vi "Flowmeter_Count and Period.vi"() -> ()   [LabVIEW 2013]
doc: "This VI counts the number of rising edges since the last sample event and measures the total period from the first to last edge in the measurement window. Divide count by period to determine the frequency."
uses:
  <vilib>/Platform/TimedLoop/XDataNode/timing_clust.ctl
  <vilib>/Platform/TimedLoop/XDataNode/nitl_modes.ctl
  <vilib>/Platform/TimedLoop/XDataNode/wakeup.ctl
  <vilib>/rvi/Emulation/niFpgaSctlEmulationGetInTimedLoop.vi
  <vilib>/rvi/Emulation/niFpgaEmulationReportErrorSimple.vi
  <vilib>/rvi/Emulation/niFpgaGetClockAttributes.vi
  <vilib>/rvi/Emulation/niFpgaCriticalErrorInLSC.vi
  <vilib>/rvi/eio/common/nirviEmuTemplateMethod_errors.vi
  Instance           2 31Saved   Count and Period (FPGA) .vi
  <vilib>/Platform/TimedLoop/XDataNode/XDataNode.xnode
  <vilib>/eio/EIONode/EIONode.xnode
  <vilib>/Platform/TimedLoop/XDataNode/XDNodeRunTimeDep.lvlib
panel:
  out "Count":u32
  out "Period":u32
  in  "Sample":bool
  in  "Polarity":bool
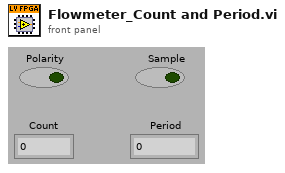
[diagram p1: front panel]
types:
  T1 = typedef "XDNodeRunTimeDep.lvlib/timing_clust.ctl" = cluster{"Expected End [f-1]":u64, "Actual End [f-1]":u64, "Finished Late? [f-1]":bool, "Expected End [i-1]":u64, "Actual End [i-1]":u64, "Finished Late? [i-1]":bool, "Expected Start [i]":u64, "Actual Start [i]":u64, "Expected Start [f]":u64, "Actual Start [f]":u64, "Source Name":string, "Structure Name":string, "Period":i64, "Deadline":i64, "Offset":i64, "Start":i64, "Priority":i32, "Timeout":i32, "Mode":T2, "Wakeup Reason":T3, "Error":errorcluster, "Source Type":string, "Secondary Source Type":string, "Global End Time":u64, "Global Start Time":u64, "Frame Duration":u64, "Iteration Duration":u64, "Assigned CPU":i32, "I/O Scan Engine Mode":u32}
  T2 = typedef "XDNodeRunTimeDep.lvlib/nitl_modes.ctl" = enum32{"No Change", "Process missed periods, maintain original phase", "Discard missed periods, maintain original phase", "Process missed periods, ignore original phase", "Discard missed periods, ignore original phase"}
  T3 = typedef "XDNodeRunTimeDep.lvlib/wakeup.ctl" = enum32{"Normal", "Aborted", "Asynchronous wakeup", "Timing source error", "Timed loop error", "Timeout"}
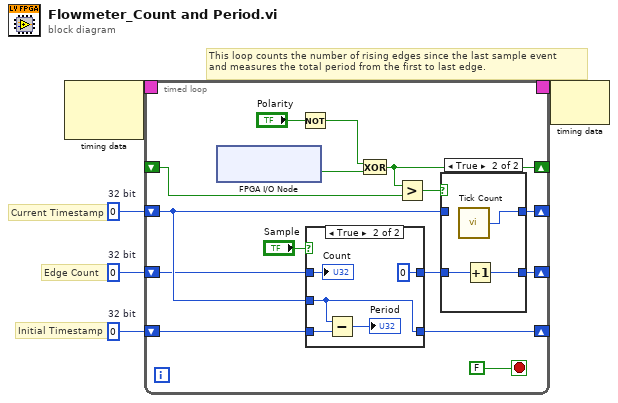
[diagram p0: block diagram]
diagram:
  w4 = u32 0  # 32 bit
  w3 = u32 0  # 32 bit
  w5 = u32 0  # 32 bit
  # "This loop counts the number of rising edges since the last sample event\nand measures the total period from the first to last edge."
  # "Initial Timestamp"
  # "Edge Count"
  # "Current Timestamp"
  n1 = node-c288() -> (w1:T1)  [unwired: 2 out]
  n2 = timed-loop {
    timing-out: [_] -> w2
    timing: w1 -> [_]
    shift-left: w4 -> [w12]
    shift-right: [w13] -> _
    shift-left: w3 -> [w14]
    shift-right: [w16] -> _
    shift-left: w5 -> [w11]
    shift-right: [w17] -> _
    shift-left: _ -> [w19]
    shift-right: [w20] -> _
    stop <- FALSE stop-if-true
    n3 = xnode "FPGA I/O Node"() -> ("Flow_meter"=w6:bool)  [unwired: 1 in, 1 out]
    n4 = Not(x="Polarity") -> (.not. x?=w7:bool)
    n5 = case shown="True" "Sample" {
      tunnel: w14 -> [_ w27]
      tunnel: [w21 w27] -> w13
      tunnel: w12 -> [w21 w26]
      tunnel: w11 -> [w22 w24]
      tunnel: [w22 u32 0 ("32 bit")] -> w10
      frame False {
      }
      frame True {
        n6 = Subtract(x=w27, y=w26) -> (x-y=→"Period":u32)
        "Count" <- w24
      }
    }
    n7 = Exclusive Or(1:w6, 2:w7) -> (0:w20:bool)
    n8 = Greater?(x=w20, y=w19) -> (0:w18:bool)
    n9 = case shown="True" w18 {
      tunnel: w10 -> [w28 w32]
      tunnel: [w28 w31] -> w17
      tunnel: [w29 w30] -> w16
      tunnel: w14 -> [w29 _]
      frame False {
      }
      frame True {
        n10 = call "Tick Count"() -> ("Tick Count(Ticks)"=w30:u32)
        n11 = Increment(x=w32) -> (x+1=w31:u32)
      }
    }
  }
  n12 = node-c288(w2) -> ()  [unwired: 1 out]
